vi "Set New Address.vi"(8 "error in (no error)":errorcluster, 10 "New Address":u8=18 format="%.0x", 11 "4ChannelSPDTRelay in":refnum<class "4ChannelSPDTRelay.lvclass">) -> (0 "error out":errorcluster, 3 "4ChannelSPDTRelay out":refnum<class "4ChannelSPDTRelay.lvclass">)   [LabVIEW 2020, in "CTI-Peripheral.lvlib" / "4ChannelSPDTRelay.lvclass"]
uses:
  4ChannelSPDTRelay.lvclass
  4ChannelSPDTRelay.lvclass/4ChannelSPDTRelay.ctl
  CTI/I2C Connection/I2C Connection.lvclass/I2C Connection.ctl
  CTI/Session/I2C Write Data.vi
  CTI/I2C Connection/I2C Connection.lvclass
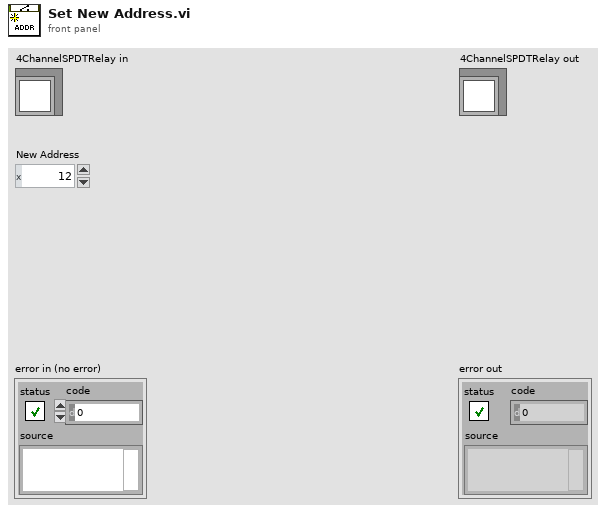
[diagram p1: front panel]
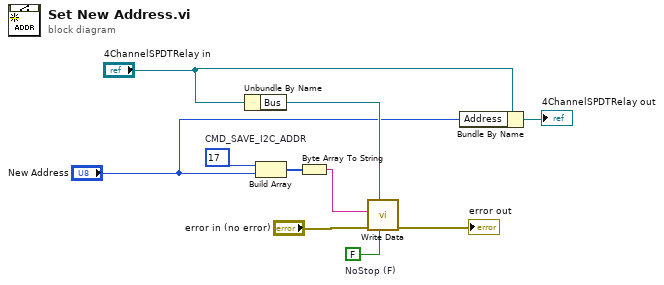
[diagram p0: block diagram]
diagram:
  w7 = FALSE  # NoStop (F)
  w6 = u8 17  # CMD_SAVE_I2C_ADDR
  n1 = Unbundle By Name("4ChannelSPDTRelay in") -> ("Bus"=w8:refnum<class "I2C Connection.lvclass">)
  n2 = Build Array(w6, "New Address") -> (w10:u8[])
  n3 = Byte Array To String(unsigned byte array=w10) -> (string=w9:string)
  n4 = call "Write Data.vi"("NoStop (F)"=w7, "I2C Connection"=w8, "error in (no error)"="error in (no error)", "Data"=w9) -> ("error out"=→"error out":errorcluster)  [unwired: 7 in]
  n5 = Bundle By Name(cluster="4ChannelSPDTRelay in", "Address"="New Address") -> (→"4ChannelSPDTRelay out":refnum<class "4ChannelSPDTRelay.lvclass">)
